vi "Reference_Inst_Info_2_string.vi"(1 "Reference instrument":T2={"high limit (10V)"=4.0, "low limit (-10V)"=0.0, "Ch No"=4, "Off ch no"=0, "Calib filename"=path "", "Ref Instrument type"=enum."Enter Value"} {"Off ch no" min=0 max=1; "Ch No" min=0 max=50; "low limit (-10V)" min=-10 max=10 format="%.1f"; "high limit (10V)" min=-10 max=10 format="%.1f"}, 2 "Reference Name":string="Instrument to calibrate") -> (0 "Setup String":string)   [LabVIEW 2011]
uses:
  Calib_setup.ctl
  Controls/Ref_Inst_type.ctl
panel:
  in  "Ref Instrument type":T1=enum."LDA"
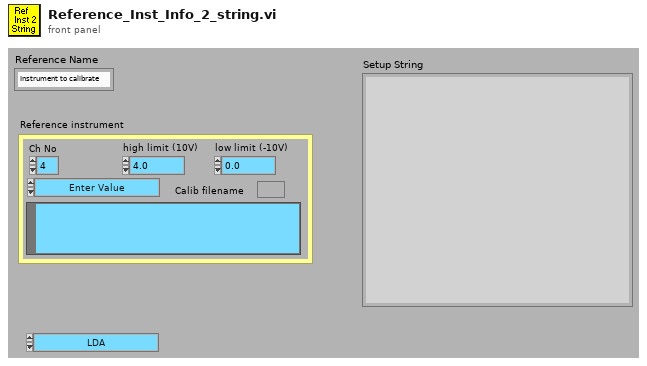
[diagram p1: front panel]
types:
  T1 = typedef "Ref_Inst_type.ctl" = enum16{"Propellor anemometer", "Pressure Transducer", "Raw voltage", "Pitot-static tube", "Preston tube", "Generic Linear", "Generic Polynomial", "Thermocouple", "LDA", "Enter Value", "ADAM Channel"}
  T2 = typedef "Calib_setup.ctl" = cluster{"high limit (10V)":sgl, "low limit (-10V)":sgl, "Ch No":i16, "Off ch no":i8, "Calib filename":path, "Ref Instrument type":T1}
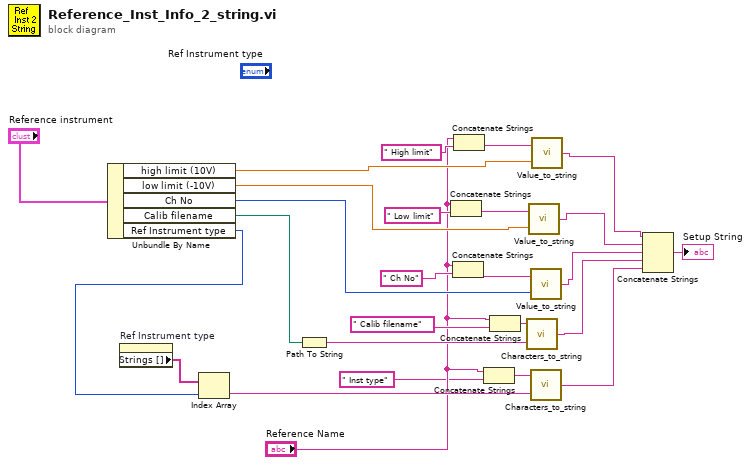
[diagram p0: block diagram]
diagram:
  n1 = Unbundle By Name("Reference instrument") -> ("high limit (10V)"=w19:sgl, "low limit (-10V)"=w18:sgl, "Ch No"=w17:i16, "Calib filename"=w13:path, "Ref Instrument type"=w11:T1)
  n2 = property on="Ref Instrument type" class="Enum (strict)"() -> ("Strings []"=w12:string[])  [unwired: 2 in, 2 out]
  n3 = Index Array(array=w12, index=w11) -> (element=w10:string)
  n4 = Path To String(path=w13) -> (string=w16:string)
  n5 = Concatenate Strings("Reference Name", " Low limit") -> (w22:string)
  n6 = Concatenate Strings("Reference Name", " Ch No") -> (w23:string)
  n7 = Concatenate Strings("Reference Name", " High limit") -> (w21:string)
  n8 = Concatenate Strings("Reference Name", " Inst type") -> (w7:string)
  n9 = Concatenate Strings("Reference Name", " Calib filename") -> (w15:string)
  n10 = call "Characters_to_string.vi"("Characters to write"=w16, "Label for characters"=w15) -> ("Output string"=w3:string)
  n11 = call "Value_to_string.vi"("Value"=w18, "Label for value"=w22) -> ("Output string"=w5:string)  [unwired: 1 in]
  n12 = call "Value_to_string.vi"("Value"=w17, "Label for value"=w23) -> ("Output string"=w4:string)  [unwired: 1 in]
  n13 = call "Characters_to_string.vi"("Characters to write"=w10, "Label for characters"=w7) -> ("Output string"=w2:string)
  n14 = call "Value_to_string.vi"("Value"=w19, "Label for value"=w21) -> ("Output string"=w6:string)  [unwired: 1 in]
  n15 = Concatenate Strings(w6, w5, w4, w3, w2) -> (→"Setup String":string)
